vi "Close P40.vi"(8 "error in (no error)":errorcluster, 11 "SSI P40 Settings In":T1={"VISA resource name"="", "Simulated?"=TRUE}) -> (0 "error out":errorcluster, 1 "Connection Error":bool, 3 "SSI P40 Settings Out":T1={"VISA resource name"="", "Simulated?"=TRUE})   [LabVIEW 2021, in "SSI P40 Pump.lvlib"]
uses:
  SSI P40 Pump.lvlib
  SSI P40 Settings Cluster.ctl
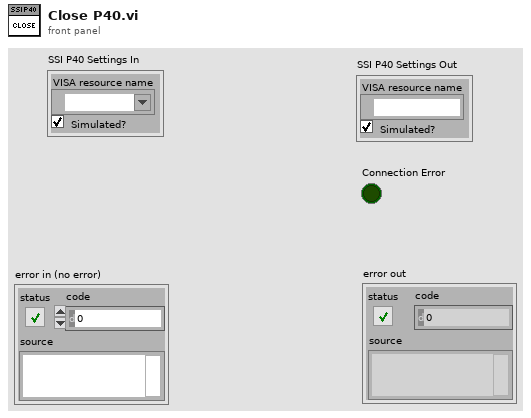
[diagram p1: front panel]
types:
  T1 = typedef "SSI P40 Pump.lvlib/SSI P40 Settings Cluster.ctl" = cluster{"VISA resource name":refnum<visa-resource-name>, "Simulated?":bool}
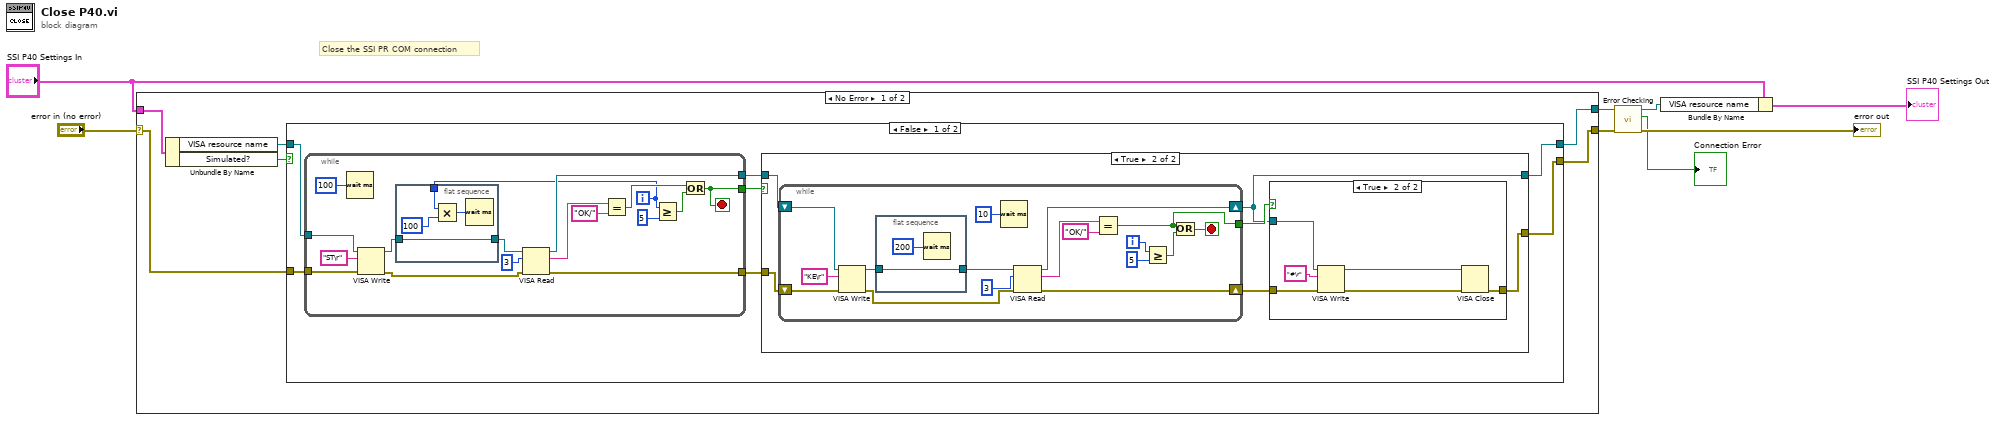
[diagram p0: block diagram]
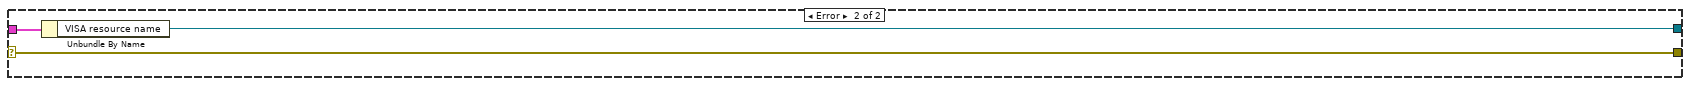
[diagram p5: hidden frame]
diagram:
  # "Close the SSI PR COM connection"
  n1 = case shown="No Error" "error in (no error)" {
    selector: "error in (no error)" -> [w14 w81]
    tunnel: "SSI P40 Settings In" -> [w10 w80]
    tunnel: [w11 w81] -> w4
    tunnel: [w9 w79] -> w5
    frame No Error {
      n2 = Unbundle By Name(w10) -> ("VISA resource name"=w12:refnum<visa-resource-name>, "Simulated?"=w13:bool)
      n3 = case shown="False" w13 {
        tunnel: w14 -> [w18 w78]
        tunnel: w12 -> [w19 w77]
        tunnel: [w21 w78] -> w11
        tunnel: [w20 w77] -> w9
        frame False {
          n4 = while {
            tunnel: w19 -> [w37]
            tunnel: w18 -> [w36]
            tunnel: [w27] -> w17
            tunnel: [w26] -> w16
            tunnel: [w23] -> w15
            i -> [w22]
            stop <- w23 stop-if-true
            n5 = Wait (ms)(milliseconds to wait=u32 100) -> ()  [unwired: 1 out]
            n6 = VISA Write(VISA resource name=w37, write buffer="ST\r", error in (no error)=w36) -> (VISA resource name out=w25:refnum<visa-resource-name>, error out=w34:errorcluster)  [unwired: 1 out]
            n7 = flat-sequence {
              tunnel: w25 -> [w42]
              tunnel: [w42] -> w24
              tunnel: w22 -> [w39]
              frame #0 {
                n8 = Multiply(x=w39, y=u32 100 ("milliseconds to wait")) -> (x*y=w41:u32)
                n9 = Wait (ms)(milliseconds to wait=w41) -> ()  [unwired: 1 out]
              }
            }
            n10 = VISA Read(VISA resource name=w24, byte count=u32 3, error in (no error)=w34) -> (VISA resource name out=w26:refnum<visa-resource-name>, read buffer=w33:string, error out=w27:errorcluster)  [unwired: 1 out]
            n11 = Equal?(x=w33, y="OK/") -> (x = y?=w31:bool)
            n12 = Greater Or Equal?(x=w22, y=5) -> (x >= y?=w29:bool)
            n13 = Or(x=w31, y=w29) -> (x .or. y?=w23:bool)
          }
          n14 = case shown="True" w15 {
            tunnel: w16 -> [w44 w46]
            tunnel: [w43 w45] -> w21
            tunnel: [w44 w48] -> w20
            tunnel: w17 -> [w43 w47]
            frame False {
            }
            frame True {
              n15 = while {
                tunnel: [w54] -> w50
                shift-right: [w65] -> w49
                shift-left: w47 -> [w60]
                shift-right: [w64] -> w48
                shift-left: w46 -> [w59]
                i -> [w52]
                stop <- w53 stop-if-true
                n16 = VISA Write(VISA resource name=w59, write buffer="KE\r", error in (no error)=w60) -> (VISA resource name out=w58:refnum<visa-resource-name>, error out=w61:errorcluster)  [unwired: 1 out]
                n17 = flat-sequence {
                  tunnel: [w68] -> w57
                  tunnel: w58 -> [w68]
                  frame #0 {
                    n18 = Wait (ms)(milliseconds to wait=u32 200) -> ()  [unwired: 1 out]
                  }
                }
                n19 = Wait (ms)(milliseconds to wait=u32 10) -> ()  [unwired: 1 out]
                n20 = VISA Read(VISA resource name=w57, byte count=u32 3, error in (no error)=w61) -> (VISA resource name out=w64:refnum<visa-resource-name>, read buffer=w62:string, error out=w65:errorcluster)  [unwired: 1 out]
                n21 = Equal?(x=w62, y="OK/") -> (x = y?=w54:bool)
                n22 = Greater Or Equal?(x=w52, y=5) -> (x >= y?=w55:bool)
                n23 = Or(x=w54, y=w55) -> (x .or. y?=w53:bool)
              }
              n24 = case shown="True" w50 {
                tunnel: w48 -> [_ w75]
                tunnel: w49 -> [w70 w74]
                tunnel: [w70 w72] -> w45
                frame False {
                }
                frame True {
                  n25 = VISA Write(VISA resource name=w75, write buffer="#\r", error in (no error)=w74) -> (VISA resource name out=w71:refnum<visa-resource-name>, error out=w73:errorcluster)  [unwired: 1 out]
                  n26 = VISA Close(VISA resource name=w71, error in (no error)=w73) -> (error out=w72:errorcluster)
                }
              }
            }
          }
        }
        frame True {
        }
      }
    }
    frame Error {
      n27 = Unbundle By Name(w80) -> ("VISA resource name"=w79:refnum<visa-resource-name>)
    }
  }
  n28 = call "Error Checking.vi"("error in (no error)"=w4, "VISA resource name"=w5) -> ("error out"=→"error out":errorcluster, "Connection Error"=→"Connection Error":bool, "VISA resource name"=w7:refnum<visa-resource-name>)  [unwired: 7 in]
  n29 = Bundle By Name(cluster="SSI P40 Settings In", "VISA resource name"=w7) -> (→"SSI P40 Settings Out":T1)
